vi "subscribe multiple data.vi"(8 "error in":errorcluster, 10 "subriscription list[]":string[](array[string]), 11 "refnum in":T1) -> (0 "error out":errorcluster, 3 "refnum in":T1)   [LabVIEW 2023, in "Publisher Subscriber.lvlib"]
uses:
  <userlib>/_Publisher Subscriber/Publisher Subscriber.lvlib
  <userlib>/_Publisher Subscriber/Controls/node refnum.ctl
  <userlib>/_Publisher Subscriber/Controls/node dvr data.ctl
  <userlib>/_Publisher Subscriber/Controls/data cluster.ctl
  <userlib>/_Publisher Subscriber/Controls/subscription bank ref.ctl
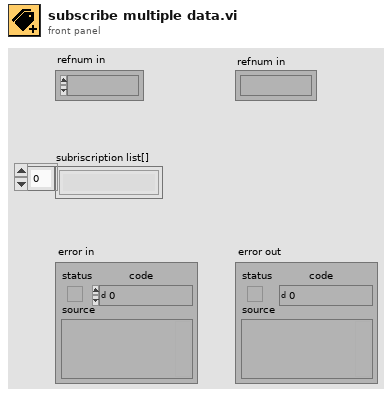
[diagram p1: front panel]
types:
  T1 = typedef "Publisher Subscriber.lvlib/node refnum.ctl" = refnum<vi>
  T2 = typedef "Publisher Subscriber.lvlib/node dvr data.ctl" = cluster{"queue ref":refnum<queue>, "Subscription Bank Ref":refnum<data-value>, "Command":string, "Data":variant, "Subscriptions []":set{string}, "Variables DVR Ref":refnum<data-value>}
  T3 = typedef "Publisher Subscriber.lvlib/subscription bank ref.ctl" = map{string, set{refnum<queue>}}
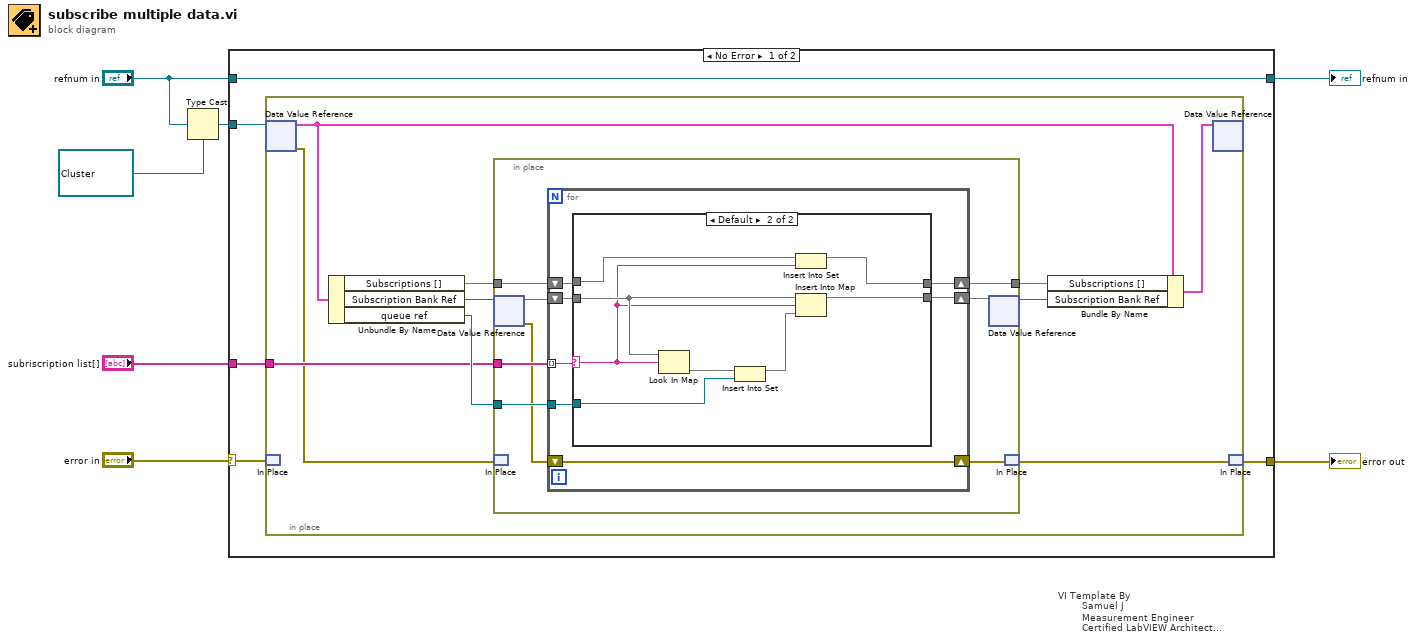
[diagram p0: block diagram]
diagram:
  n1 = Type Cast(type=refnum<data-value> refnum ("data value reference"), x="refnum in") -> (*(type *) &x=w4:refnum<data-value>)
  n2 = case "VI Template By\n        Samuel J\n        Measurement Engineer\n        Certified LabVIEW Architect\n        Vestas Technology R&D Chennai" shown="No Error" "error in" {
    selector: "error in" -> [w9 w49]
    tunnel: [w8 w49] -> w6
    tunnel: w4 -> [w10 _]
    tunnel: [w12 w48] -> w3
    tunnel: "refnum in" -> [w12 w48]
    tunnel: "subriscription list[]" -> [w11 _]
    frame No Error {
      n3 = in-place {
        in-place-border: w11 -> [w16]
        n4 = in-place-dvr #1(w10) -> (w21:T2, w15:errorcluster)
        n5 = in-place-match #2(w9) -> ()  [unwired: 1 out]
        n6 = Unbundle By Name(w21) -> ("Subscriptions []"=w17:set{string}, "Subscription Bank Ref"=w20:refnum<data-value>, "queue ref"=w18:refnum<queue>)
        n7 = in-place {
          in-place-border: w16 -> [w27]
          in-place-border: w18 -> [w28]
          in-place-border: w17 -> [w26]
          in-place-border: [w25] -> w13
          n8 = in-place-dvr #3(w20) -> (w30:T3, w23:errorcluster)
          n9 = in-place-match #4(w15) -> ()  [unwired: 1 out]
          n10 = for {
            tunnel: w28 -> [w37]
            tunnel: w27 -> [w33] mode=indexing
            shift-right: [w32] -> w29
            shift-left: w30 -> [w34]
            shift-right: [w35] -> w25
            shift-left: w26 -> [w36]
            shift-right: [w31] -> w24
            shift-left: w23 -> [w31]
            n11 = case shown="Default" w33 {
              selector: w33 -> [_ w41]
              tunnel: w34 -> [w38 w46]
              tunnel: [w38 w45] -> w32
              tunnel: w37 -> [_ w44]
              tunnel: w36 -> [w39 w42]
              tunnel: [w39 w40] -> w35
              frame "" {
              }
              frame Default {
                n12 = Look In Map(map=w46, key=w41) -> (value=w47:set{refnum<queue>})  [unwired: 1 in, 1 out]
                n13 = Insert Into Set(10:w44, 11:w47) -> (3:w43:set{refnum<queue>})  [unwired: 1 out]
                n14 = Insert Into Set(10:w41, 11:w42) -> (3:w40:set{string})  [unwired: 1 out]
                n15 = Insert Into Map(map in=w46, key=w41, value=w43) -> (map out=w45:T3)  [unwired: 2 out]
              }
            }
          }
          n16 = in-place-dvr #3(w29) -> (w19:refnum<data-value>)  [unwired: 1 out]
          n17 = in-place-match #4(w24) -> (w14:errorcluster)
        }
        n18 = Bundle By Name(cluster=w21, "Subscriptions []"=w13, "Subscription Bank Ref"=w19) -> (w22:T2)
        n19 = in-place-dvr #1(w22) -> ()  [unwired: 2 out]
        n20 = in-place-match #2(w14) -> (w8:errorcluster)
      }
    }
    frame Error {
    }
  }
  "error out" <- w6
  "refnum in" <- w3
